vi "Selu.vi"(2 "Z":dbl) -> (0 "Selu(Z)":dbl)   [LabVIEW 2020]
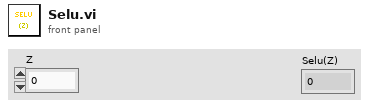
[diagram p1: front panel]
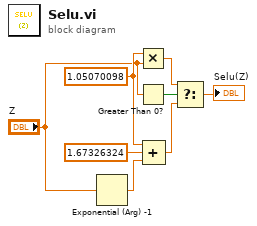
[diagram p0: block diagram]
diagram:
  w4 = 1.05070098 ("x")
  n1 = Exponential (Arg) -1(1:"Z") -> (0:w2:dbl)
  n2 = Multiply(x=w4, y="Z") -> (x*y=w6:dbl)
  n3 = Greater Than 0?(x="Z") -> (x > 0?=w7:bool)
  n4 = Compound Arithmetic op=ADD(w4, 1.67326324 ("value"), w2) -> (w5:dbl)
  n5 = Select(t=w6, s=w7, f=w5) -> (s? t:f=→"Selu(Z)":dbl)
